vi "PhotonUtils_TestGetDateTime.vi"(8 "error in (no error)":errorcluster) -> (0 "error out":errorcluster, 1 "LV Date Time Cnv":u64, 2 "DateTime":u64, 3 "TimeStamp":u64)   [LabVIEW 2019]
uses:
  Program Files/National Instruments/LabVIEW 2019/Targets/NI/RT/vi.lib/ni_emb.dll
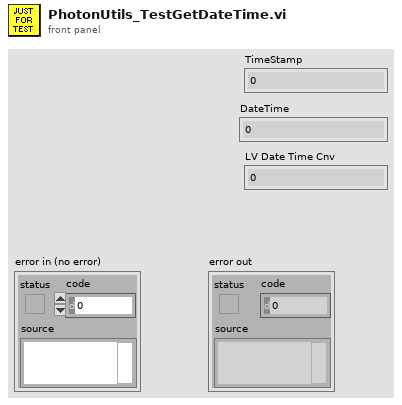
[diagram p1: front panel]
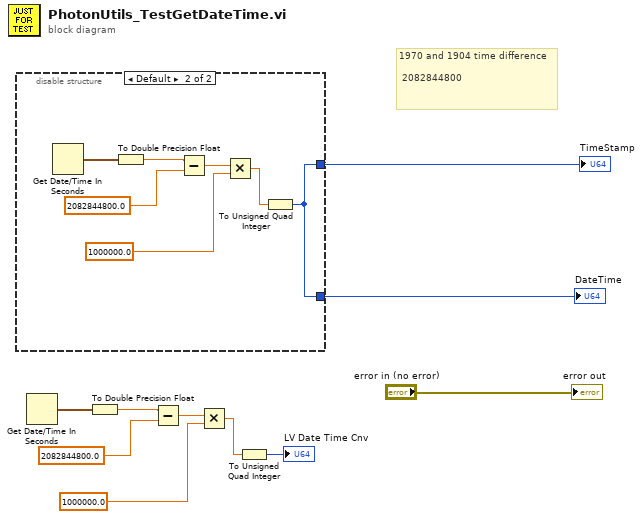
[diagram p0: block diagram]
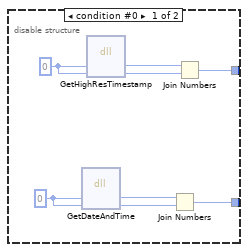
[diagram p2: hidden frame]
diagram:
  # "1970 and 1904 time difference\n\n 2082844800"
  n1 = disable-structure shown="Default" {
    disable-tunnel: [w12 w19] -> w9
    disable-tunnel: [w11 w19] -> w8
    frame condition #0 {
      w14 = u32 0 ("InH")
      w13 = u32 0 ("InH")
      n2 = dll-call lib="C:/Program Files/National Instruments/LabVIEW 2019/Targets/NI/RT/vi.lib/ni_emb.*" fn="GetDateAndTime"("tsH"=w14, "tsL"=w14) -> ("tsH"=w17:u32, "tsL"=w18:u32)  [unwired: 3 in, 3 out]
      n3 = dll-call lib="C:/Program Files/National Instruments/LabVIEW 2019/Targets/NI/RT/vi.lib/ni_emb.*" fn="GetHighResTimestamp"("tsH"=w13, "tsL"=w13) -> ("tsH"=w15:u32, "tsL"=w16:u32)  [unwired: 3 in, 3 out]
      n4 = Join Numbers(hi=w17, lo=w18) -> ((hi.lo)=w12:u64)
      n5 = Join Numbers(hi=w15, lo=w16) -> ((hi.lo)=w11:u64)
    }
    frame condition #1 (active) {
      n6 = Get Date/Time In Seconds() -> (seconds since 1Jan1904=w25:timestamp)
      n7 = To Double Precision Float(number=w25) -> (double precision float=w24:dbl)
      n8 = Subtract(x=w24, y=2082844800.0) -> (x-y=w22:dbl)
      n9 = Multiply(x=w22, y=1000000.0) -> (x*y=w20:dbl)
      n10 = To Unsigned Quad Integer(1:w20) -> (0:w19:u64)
    }
  }
  "TimeStamp" <- w8
  "DateTime" <- w9
  n11 = Get Date/Time In Seconds() -> (seconds since 1Jan1904=w7:timestamp)
  n12 = To Double Precision Float(number=w7) -> (double precision float=w6:dbl)
  n13 = Subtract(x=w6, y=2082844800.0) -> (x-y=w4:dbl)
  n14 = Multiply(x=w4, y=1000000.0) -> (x*y=w2:dbl)
  n15 = To Unsigned Quad Integer(1:w2) -> (0:→"LV Date Time Cnv":u64)
  "error out" <- "error in (no error)"
